vi "Command Type.vi"(11 "Add To Var Command Config in":refnum<class "Add To Var Command Config.lvclass">) -> (2 "Command Type":T1)   [LabVIEW 2020, in "VolatusSeqConfig.lvlib" / "Add To Var Command Config.lvclass"]
uses:
  Add To Var Command Config.lvclass
  Add To Var Command Config.lvclass/Add To Var Command Config.ctl
  Command Type.ctl
  VolatusSeqConfig.lvlib
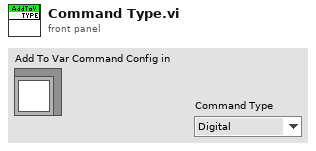
[diagram p1: front panel]
types:
  T1 = typedef "VolatusSeqConfig.lvlib/Command Type.ctl" = enum16{"Digital", "Numeric", "Transition", "Stop", "StartLog", "StopLog", "Start", "Event", "Error", "HTTP", "ResetVar", "IncVar", "DecVar", "SaveVar", "LoadVar", "AddVar", "SubVar", "SetVar", "AddToVar"}
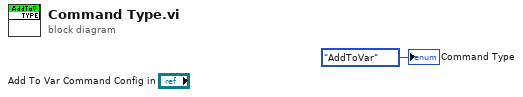
[diagram p0: block diagram]
diagram:
  "Command Type" <- Command_Type."AddToVar" ("Command Type")
